vi "CVTEngineUI.vi"() -> ()   [LabVIEW 2013, in "CVT Engine Editor.lvclass"]
uses:
  CVT Engine Editor.lvclass
  <vilib>/NI/Configuration Framework/Node/NodeRef.ctl
  <vilib>/NI/Configuration Framework/Node/NISE_CEF_Node.lvclass
  <vilib>/NI/AMC/Message Queue.ctl
  <vilib>/NI/AMC/Message.ctl
  <vilib>/NI/Tools/Keyed Array/KeyedArray.ctl
  <vilib>/NI/Configuration Framework/Node/UserEventRef.ctl
  <vilib>/NI/Configuration Framework/Controls/EventCluster.ctl
  <vilib>/NI/Tag Bus Data Framework/Configuration Editor/Classes/Engine Parent/Engine Parent Editor Node.lvclass
  <vilib>/NI/AMC/Create Single Message.vi
  <vilib>/NI/AMC/Update Message Routing Info.vi
  <vilib>/NI/Configuration Framework/serializable configuration/get alias.vi
  <vilib>/NI/AMC/Send Message.vi
  <vilib>/NI/Configuration Framework/serializable configuration/set alias.vi
  <vilib>/NI/AMC/AMC.lvlib
  <vilib>/NI/Tools/Keyed Array/Tools_KeyedArray.lvlib
  <vilib>/NI/Configuration Framework/NISE_CEF_TreeControl.lvlib
panel:
  in  "user event":T1
  in  "main queue":T2
  in  "Name":string
  in  "node ref":T3
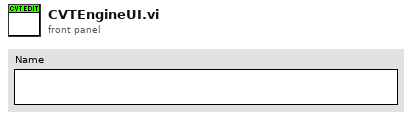
[diagram p1: front panel]
types:
  T1 = typedef "NISE_CEF_Node.lvclass/UserEventRef.ctl" = refnum<user-event>
  T2 = typedef "AMC.lvlib/Message Queue.ctl" = refnum<queue>
  T3 = typedef "NISE_CEF_Node.lvclass/NodeRef.ctl" = refnum<data-value>
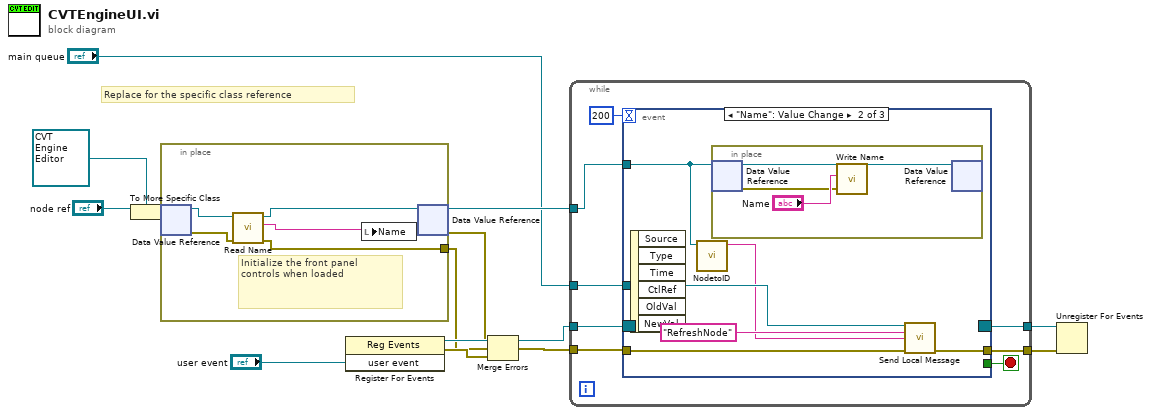
[diagram p0: block diagram]
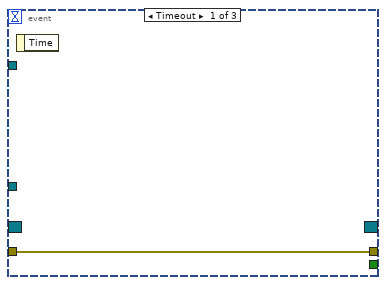
[diagram p2: hidden frame]
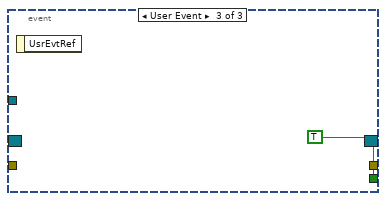
[diagram p3: hidden frame]
diagram:
  # "Replace for the specific class reference"
  n1 = To More Specific Class(target class=refnum<data-value> refnum ("data value reference"), reference="node ref") -> (specific class reference=w5:refnum<data-value>)  [unwired: 1 in, 1 out]
  n2 = in-place {
    in-place-border: [w14] -> w1
    # "Initialize the front panel  controls when loaded"
    n3 = in-place-dvr #1(w5) -> (w18:refnum<class "CVT Engine Editor.lvclass">, w17:errorcluster)
    n4 = call <vilib>:"Read Name.vi"("error in"=w17, "Engine in"=w18) -> ("error out"=w14:errorcluster, "Name"=w16:string, "Engine out"=w15:refnum<class "CVT Engine Editor.lvclass">)  [unwired: 7 in]
    n5 = local write "Name"(w16) -> ()
    n6 = in-place-dvr #1(w15) -> (w13:refnum<data-value>, w2:errorcluster)
  }
  n7 = register-events("user event") -> (reference out=w10:refnum<event-registration>, error out=w7:errorcluster)  [unwired: 2 in]
  n8 = Merge Errors(w2, w1, w7) -> (w3:errorcluster)
  n9 = while {
    tunnel: w13 -> [w26]
    tunnel: "main queue" -> [w25]
    tunnel: w10 -> [w23]
    tunnel: [w22] -> w9
    tunnel: [w20] -> w8
    tunnel: w3 -> [w19]
    stop <- w21 stop-if-true
    n10 = event shown="[1] \"Name\": Value Change" {
      selector: w23 -> [_ _ _]
      dyn-events: [_ _ _] -> w22
      timeout: 200 -> [_ _ _]
      tunnel: w26 -> [_ w31 _]
      tunnel: w25 -> [_ w32 _]
      tunnel: [_ _ TRUE] -> w21
      tunnel: [w27 w29 _] -> w20
      tunnel: w19 -> [w27 w28 _]
      event Timeout {
        n11 = event-data() -> ()  [unwired: 1 in, 1 out]
      }
      event "Name": Value Change {
        n12 = event-data() -> ()  [unwired: 1 in, 6 out]
        n13 = call <vilib>:"NodetoID.vi"("node ref"=w31) -> ("ID"=w30:string)  [unwired: 9 in, 1 out]
        n14 = in-place {
          n15 = in-place-dvr #2(w31) -> (w37:refnum<class "CVT Engine Editor.lvclass">, w35:errorcluster)
          n16 = call <vilib>:"Write Name.vi"("error in"=w35, "Name"="Name", "Engine in"=w37) -> ("Engine out"=w34:refnum<class "CVT Engine Editor.lvclass">)  [unwired: 7 in, 1 out]
          n17 = in-place-dvr #2(w34) -> ()  [unwired: 2 out]
        }
        n18 = call <vilib>:"Send Local Message.vi"("message queue in"=w32, "message name"="RefreshNode" ("Message Name"), "message value"=w30, "error in"=w28) -> ("error out"=w29:errorcluster)  [unwired: 9 in, 2 out]
      }
      event User Event {
        n19 = event-data() -> ()  [unwired: 1 in, 1 out]
      }
    }
  }
  n20 = Unregister For Events(event registration refnum=w9, error in=w8) -> ()  [unwired: 1 out]
